vi "mqtt payload to double.vi"(2 "double type":dbl, 7 "MQTT payload":string="MQTT payload") -> (8 "double":dbl, 13 "error out":errorcluster)   [LabVIEW 2017]
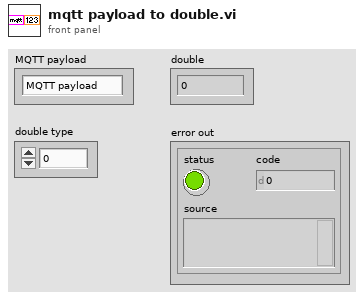
[diagram p1: front panel]
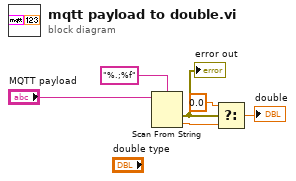
[diagram p0: block diagram]
diagram:
  n1 = Scan From String(format string="%.;%f", input string="MQTT payload") -> (error out=w4:errorcluster, output 1=w2:dbl)  [unwired: 3 in, 2 out]
  "error out" <- w4
  n2 = Select(t=0.0, s=w4, f=w2) -> (s? t:f=→"double":dbl)
